vi "CRYCurve Cut to Range.vi"(8 "Axis type (Lin)":u16(ring)=1 items=["Log", "Lin"], 9 "Range variable (x)":enum16{"x", "y", "z"}(ring), 10 "Search range":string[](array[string]), 11 "Curve in":cluster{"x":dbl, "y":dbl, "z":dbl}[](array[cluster]) {"z" format="%.2f"; "y" format="%.2f"; "x" format="%.2f"}) -> (3 "Cut curve out":cluster{"x":dbl, "y":dbl, "z":dbl}[](array[cluster]) {"z" format="%.2f"; "y" format="%.2f"; "x" format="%.2f"})   [LabVIEW 2013]
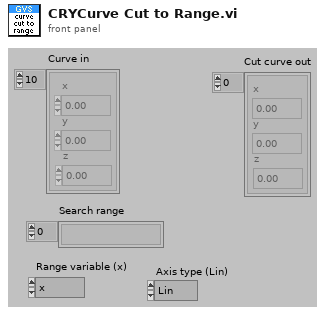
[diagram p1: front panel]
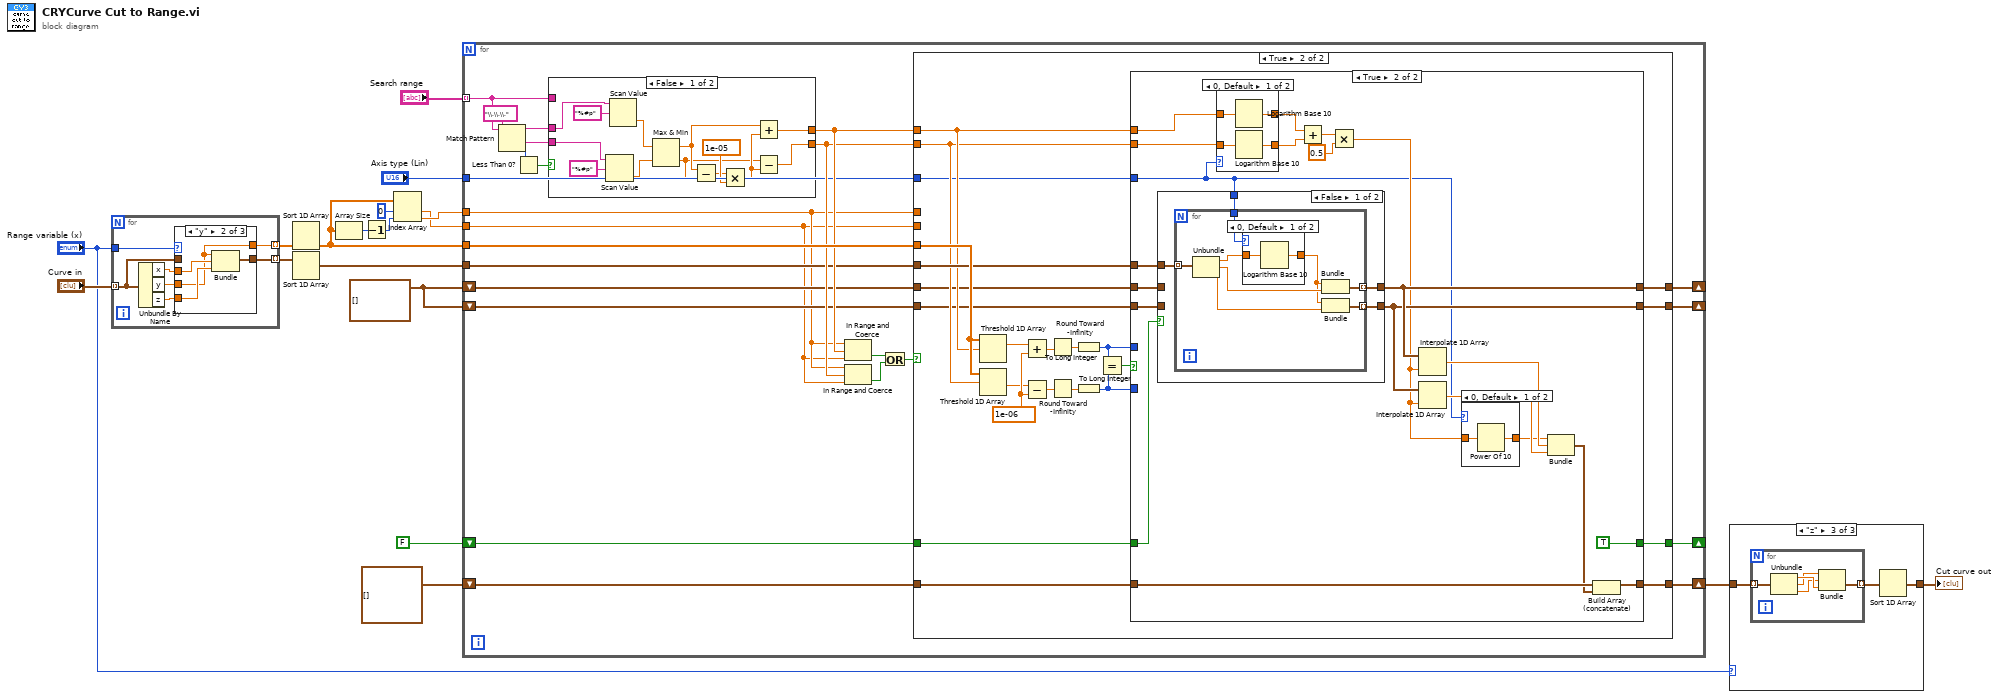
[diagram p0: block diagram]
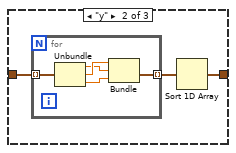
[diagram p3: hidden frame]
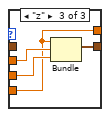
[diagram p5: hidden frame]
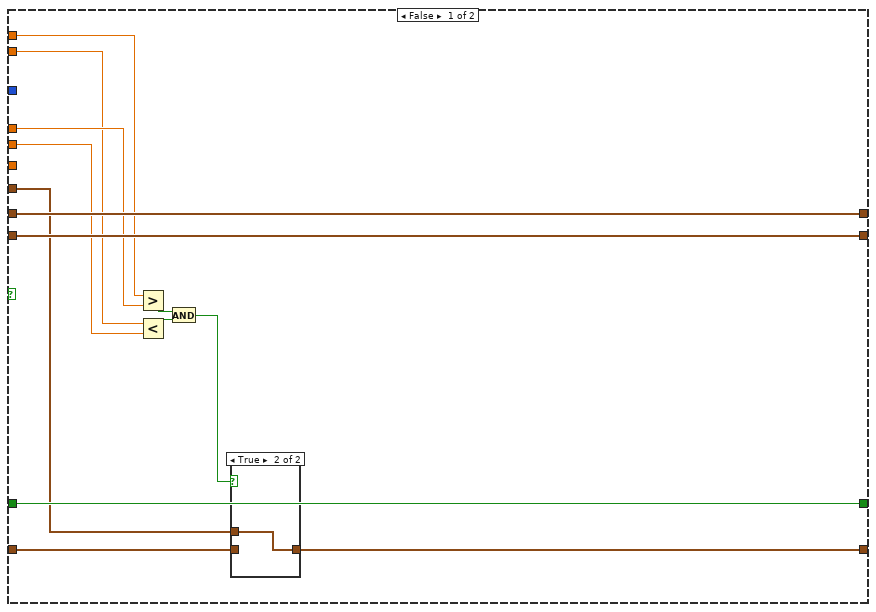
[diagram p6: hidden frame]
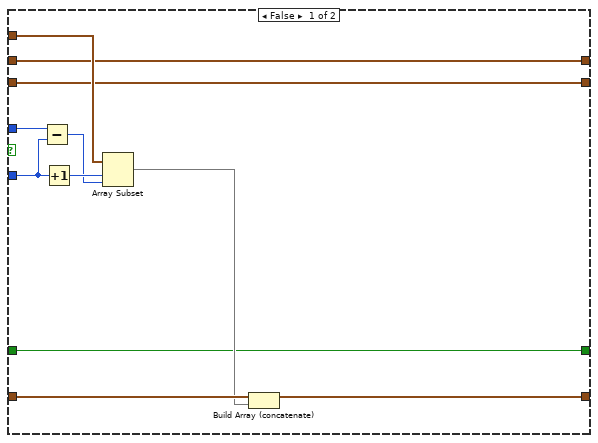
[diagram p8: hidden frame]
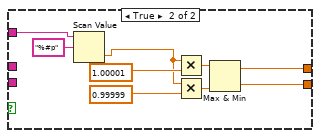
[diagram p13: hidden frame]
diagram:
  w7 = cluster{"z":dbl, dbl}[] []
  n1 = for {
    tunnel: "Curve in" -> [w21] mode=indexing
    tunnel: "Range variable (x)" -> [w25]
    tunnel: [w20] -> w14 mode=indexing
    tunnel: [w19] -> w10 mode=indexing
    n2 = Unbundle By Name(w21) -> ("x"=w24:dbl, "y"=w23:dbl, "z"=w22:dbl)
    n3 = case shown="\"y\"" w25 {
      tunnel: w24 -> [w26 w30 w35]
      tunnel: w23 -> [_ w28 w34]
      tunnel: w22 -> [_ w29 w32]
      tunnel: [w27 w31 w33] -> w19
      tunnel: w21 -> [w27 _ _]
      tunnel: [w26 w28 w32] -> w20
      frame "x", Default {
      }
      frame "y" {
        n4 = Bundle("y"=w28, "x"=w30, "z"=w29) -> (w31:cluster{"y":dbl, "x":dbl, "z":dbl})  [unwired: 1 out]
      }
      frame "z" {
        n5 = Bundle("z"=w32, "x"=w35, "y"=w34) -> (w33:cluster{"z":dbl, "x":dbl, "y":dbl})  [unwired: 1 out]
      }
    }
  }
  n6 = Sort 1D Array(array=w14) -> (sorted array=w11:dbl[])
  n7 = Sort 1D Array(array=w10) -> (sorted array=w9:cluster{"z":dbl, "x":dbl, "y":dbl}[])
  n8 = Array Size(array=w11) -> (size(s)=w13:i32)
  n9 = Decrement(x=w13) -> (x-1=w12:i32)
  n10 = Index Array(array=w11, index #1=0 ("Index"), index #2=w12) -> (element #1=w2:dbl, element #2=w3:dbl)
  n11 = for {
    tunnel: "Search range" -> [w54] mode=indexing
    tunnel: w3 -> [w38]
    tunnel: w2 -> [w37]
    tunnel: w11 -> [w48]
    shift-right: [w49] -> w5
    shift-left: cluster{"x":dbl, "y":dbl, "z":dbl}[] [] -> [w50]
    tunnel: w9 -> [w45]
    shift-right: [w41] -> _
    shift-left: w7 -> [w44]
    shift-right: [w40] -> _
    shift-left: w7 -> [w43]
    shift-right: [w39] -> _
    shift-left: FALSE -> [w42]
    tunnel: "Axis type (Lin)" -> [w36]
    n12 = Match Pattern(string=w54, regular expression="\\.\\.\\.") -> (before substring=w55:string, after substring=w56:string, offset past match=w58:i32)  [unwired: 2 out]
    n13 = Less Than 0?(x=w58) -> (x < 0?=w57:bool)
    n14 = case shown="False" w57 {
      tunnel: w56 -> [w157 _]
      tunnel: w55 -> [w160 _]
      tunnel: w54 -> [_ w170]
      tunnel: [w164 w173] -> w47
      tunnel: [w165 w172] -> w46
      frame False {
        n15 = Scan Value(string=w157, format string="%#p") -> (value=w156:dbl)  [unwired: 1 in, 1 out]
        n16 = Scan Value(string=w160, format string="%#p") -> (value=w159:dbl)  [unwired: 1 in, 1 out]
        n17 = Max & Min(x=w159, y=w156) -> (max(x,y)=w163:dbl, min(x,y)=w162:dbl)
        n18 = Subtract(x=w163, y=w162) -> (x-y=w167:dbl)
        n19 = Multiply(x=w167, y=1e-05) -> (x*y=w166:dbl)
        n20 = Add(x=w163, y=w166) -> (x+y=w164:dbl)
        n21 = Subtract(x=w162, y=w166) -> (x-y=w165:dbl)
      }
      frame True {
        n22 = Scan Value(string=w170, format string="%#p") -> (value=w169:dbl)  [unwired: 1 in, 1 out]
        n23 = Multiply(x=w169, y=1.00001) -> (x*y=w175:dbl)
        n24 = Multiply(x=w169, y=0.99999) -> (x*y=w174:dbl)
        n25 = Max & Min(x=w175, y=w174) -> (max(x,y)=w173:dbl, min(x,y)=w172:dbl)
      }
    }
    n26 = In Range and Coerce(upper limit=w38, x=w47, lower limit=w37) -> (In Range?=w53:bool)  [unwired: 1 out]
    n27 = In Range and Coerce(upper limit=w38, x=w46, lower limit=w37) -> (In Range?=w52:bool)  [unwired: 1 out]
    n28 = Or(x=w53, y=w52) -> (x .or. y?=w51:bool)
    n29 = case shown="True" w51 {
      tunnel: w50 -> [w63 w90]
      tunnel: [w62 w89] -> w49
      tunnel: w48 -> [_ w97]
      tunnel: w47 -> [w69 w88]
      tunnel: w46 -> [w67 w87]
      tunnel: w45 -> [w61 w93]
      tunnel: w44 -> [w72 w86]
      tunnel: w43 -> [w71 w85]
      tunnel: w42 -> [w70 w84]
      tunnel: [w72 w83] -> w41
      tunnel: [w71 w82] -> w40
      tunnel: [w70 w81] -> w39
      tunnel: w38 -> [w68 _]
      tunnel: w37 -> [w66 _]
      tunnel: w36 -> [_ w75]
      frame False {
        n30 = Greater?(x=w69, y=w68) -> (0:w65:bool)
        n31 = Less?(x=w67, y=w66) -> (x < y?=w64:bool)
        n32 = And(x=w65, y=w64) -> (x .and. y?=w60:bool)
        n33 = case shown="True" w60 {
          tunnel: w63 -> [w73 _]
          tunnel: [w73 w74] -> w62
          tunnel: w61 -> [_ w74]
          frame False {
          }
          frame True {
          }
        }
      }
      frame True {
        w80 = 1e-06
        n34 = Threshold 1D Array(2:w88, 3:w97) -> (0:w78:dbl)  [unwired: 1 out]
        n35 = Threshold 1D Array(2:w87, 3:w97) -> (0:w79:dbl)  [unwired: 1 out]
        n36 = Add(x=w78, y=w80) -> (x+y=w77:dbl)
        n37 = Subtract(x=w79, y=w80) -> (x-y=w76:dbl)
        n38 = Round Toward -Infinity(1:w77) -> (0:w95:dbl)
        n39 = Round Toward -Infinity(1:w76) -> (0:w96:dbl)
        n40 = To Long Integer(number=w95) -> (32bit integer=w92:i32)
        n41 = To Long Integer(number=w96) -> (32bit integer=w91:i32)
        n42 = Equal?(x=w92, y=w91) -> (x = y?=w94:bool)
        n43 = case shown="True" w94 {
          tunnel: w93 -> [w105 w123]
          tunnel: w92 -> [w108 _]
          tunnel: w91 -> [w107 _]
          tunnel: w90 -> [w103 w120]
          tunnel: [w102 w118] -> w89
          tunnel: w88 -> [_ w113]
          tunnel: w87 -> [_ w112]
          tunnel: w86 -> [w100 w126]
          tunnel: w85 -> [w99 w125]
          tunnel: w84 -> [w98 w127]
          tunnel: [w100 w122] -> w83
          tunnel: [w99 w121] -> w82
          tunnel: [w98 TRUE] -> w81
          tunnel: w75 -> [_ w109]
          frame False {
            n44 = Subtract(x=w108, y=w107) -> (x-y=w104:i32)
            n45 = Increment(x=w107) -> (x+1=w106:i32)
            n46 = Array Subset(array=w105, index=w106, length=w104) -> (w101:cluster{"z":dbl, "x":dbl, "y":dbl}[])
            n47 = Build Array (concatenate)(w103, w101) -> (w102:cluster{"z":dbl, "x":dbl, "y":dbl}[])
          }
          frame True {
            n48 = case shown="False" w127 {
              tunnel: w126 -> [_ w155]
              tunnel: w125 -> [_ w154]
              tunnel: [w141 w155] -> w122
              tunnel: [w140 w154] -> w121
              tunnel: w123 -> [w142 _]
              tunnel: w109 -> [w139 _]
              frame False {
                n49 = for {
                  tunnel: w142 -> [w150] mode=indexing
                  tunnel: [w149] -> w141 mode=indexing
                  tunnel: [w148] -> w140 mode=indexing
                  tunnel: w139 -> [w143]
                  n50 = Unbundle(w150) -> ("z"=w145:dbl, "x"=w147:dbl, "y"=w146:dbl)
                  n51 = case shown="0, Default" w143 {
                    tunnel: w145 -> [w152 w153]
                    tunnel: [w151 w153] -> w144
                    frame 0, Default {
                      n52 = Logarithm Base 10(1:w152) -> (0:w151:dbl)
                    }
                    frame 1 {
                    }
                  }
                  n53 = Bundle("z"=w144, "x"=w147) -> (w149:cluster{"z":dbl, "x":dbl})  [unwired: 1 out]
                  n54 = Bundle("z"=w144, "y"=w146) -> (w148:cluster{"z":dbl, "y":dbl})  [unwired: 1 out]
                }
              }
              frame True {
              }
            }
            n55 = case shown="0, Default" w109 {
              tunnel: w113 -> [w133 w135]
              tunnel: [w132 w135] -> w111
              tunnel: [w131 w134] -> w110
              tunnel: w112 -> [w130 w134]
              frame 0, Default {
                n56 = Logarithm Base 10(1:w133) -> (0:w132:dbl)
                n57 = Logarithm Base 10(1:w130) -> (0:w131:dbl)
              }
              frame 1 {
              }
            }
            n58 = Add(x=w111, y=w110) -> (x+y=w129:dbl)
            n59 = Multiply(x=w129, y=0.5) -> (x*y=w115:dbl)
            n60 = Interpolate 1D Array(1:w115, 2:w122) -> (0:w117:dbl)
            n61 = Interpolate 1D Array(1:w115, 2:w121) -> (0:w116:dbl)
            n62 = case shown="0, Default" w109 {
              tunnel: w115 -> [w137 w138]
              tunnel: [w136 w138] -> w114
              frame 0, Default {
                n63 = Power Of 10(x=w137) -> (10^x=w136:dbl)
              }
              frame 1 {
              }
            }
            n64 = Bundle(w114, w117, w116) -> (w119:cluster{dbl, dbl, dbl})  [unwired: 1 out]
            n65 = Build Array (concatenate)(w120, w119) -> (w118:cluster{"x":dbl, "y":dbl, "z":dbl}[])
          }
        }
      }
    }
  }
  n66 = case shown="\"z\"" "Range variable (x)" {
    tunnel: w5 -> [w178 w181 w189]
    tunnel: [w178 w179 w187] -> w4
    frame "x", Default {
    }
    frame "y" {
      n67 = for {
        tunnel: w181 -> [w186] mode=indexing
        tunnel: [w182] -> w180 mode=indexing
        n68 = Unbundle(w186) -> ("x"=w184:dbl, "y"=w185:dbl, "z"=w183:dbl)
        n69 = Bundle("y"=w185, "x"=w184, "z"=w183) -> (w182:cluster{"y":dbl, "x":dbl, "z":dbl})  [unwired: 1 out]
      }
      n70 = Sort 1D Array(array=w180) -> (sorted array=w179:cluster{"y":dbl, "x":dbl, "z":dbl}[])
    }
    frame "z" {
      n71 = for {
        tunnel: w189 -> [w194] mode=indexing
        tunnel: [w193] -> w188 mode=indexing
        n72 = Unbundle(w194) -> ("x"=w192:dbl, "y"=w191:dbl, "z"=w190:dbl)
        n73 = Bundle("y"=w191, "z"=w190, "x"=w192) -> (w193:cluster{"y":dbl, "z":dbl, "x":dbl})  [unwired: 1 out]
      }
      n74 = Sort 1D Array(array=w188) -> (sorted array=w187:cluster{"y":dbl, "z":dbl, "x":dbl}[])
    }
  }
  "Cut curve out" <- w4
